vi "Get Path.vi"(8 "error in (no error)":errorcluster) -> (0 "error out":errorcluster, 3 "Path":path)   [LabVIEW 2017, in "Log.lvclass"]
uses:
  Log.lvclass
  Log_Facilities.ctl
  Log_Facility.ctl
  Log_Level.ctl
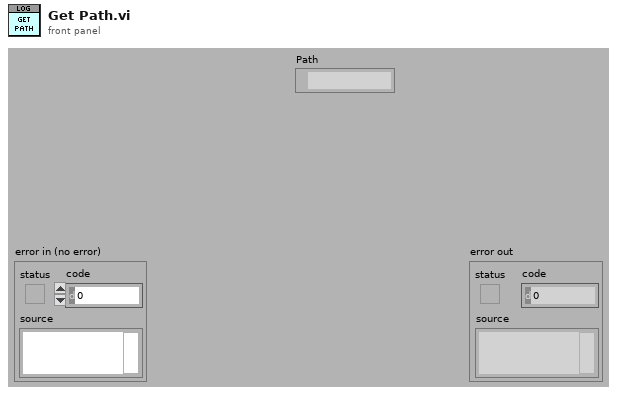
[diagram p1: front panel]
types:
  T1 = typedef "Log.lvclass/Log_Facility.ctl" = cluster{"Path":path, "Ref":refnum<file>, "Level":T2}
  T2 = typedef "Log.lvclass/Log_Level.ctl" = enum16{"none", "info", "trace", "warn", "error", "fatal"}
  T3 = typedef "Log.lvclass/Log_Facilities.ctl" = string
  T4 = typedef "Log.lvclass/ObjectAttributes.ctl" = cluster{"Level":T2, "Facilities":variant, "Event":refnum<user-event>}
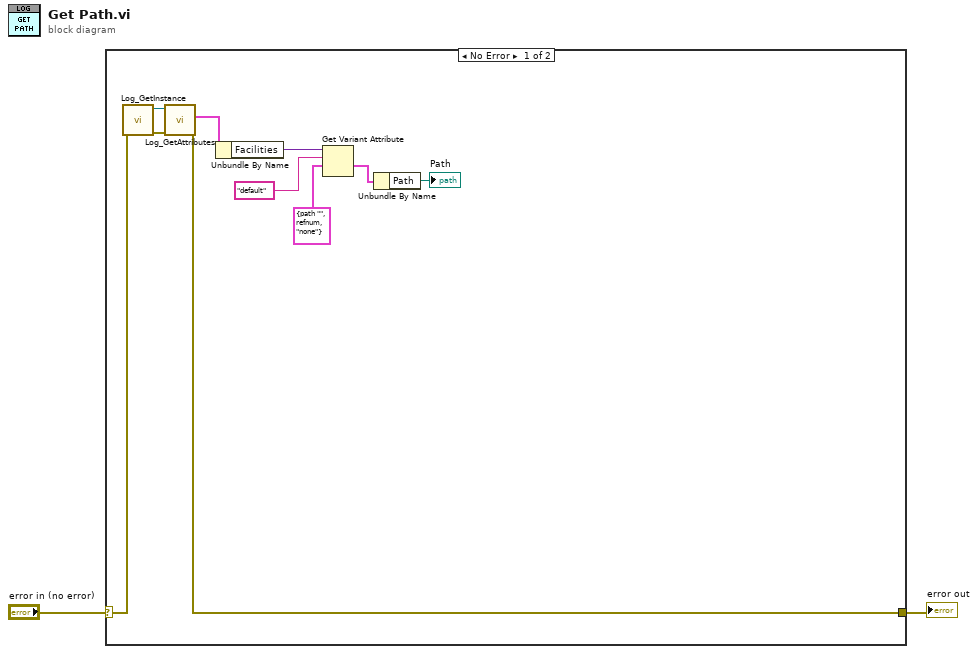
[diagram p0: block diagram]
diagram:
  n1 = case shown="No Error" "error in (no error)" {
    selector: "error in (no error)" -> [w9 w13]
    tunnel: [w11 w13] -> w1
    frame No Error {
      n2 = call "Log_GetInstance.vi"("error in (no error)"=w9) -> ("error out"=w8:errorcluster, "reference out"=w10:refnum<class "Log.lvclass">)  [unwired: 6 in, 3 out]
      n3 = call "Log_GetAttributes.vi"("error in (no error)"=w8, "reference in"=w10) -> ("error out"=w11:errorcluster, "Data"=w12:T4)  [unwired: 6 in, 2 out]
      n4 = Unbundle By Name(w12) -> ("Facilities"=w7:variant)
      n5 = Get Variant Attribute(Variant=w7, name=T3 "default" ("Name"), default value (empty Variant)=T1 {"Path"=path "", "Ref"=refnum, "Level"=enum."none"} ("Cluster")) -> (value=w4:T1)  [unwired: 1 in, 3 out]
      n6 = Unbundle By Name(w4) -> ("Path"=→"Path":path)
    }
    frame Error {
    }
  }
  "error out" <- w1
